vi "Array Functions Part 2.vi"() -> ()   [LabVIEW 2015]
panel:
  out "Initialized + Replaced Result":bool[](array[boolean])
  out "Build Array Result":dbl[](array[numeric])
  out "Array Subset Result":dbl[](array[numeric])
  out "min index(es)":i32
  out "min value":dbl
  out "max index(es)":i32
  out "max value":dbl
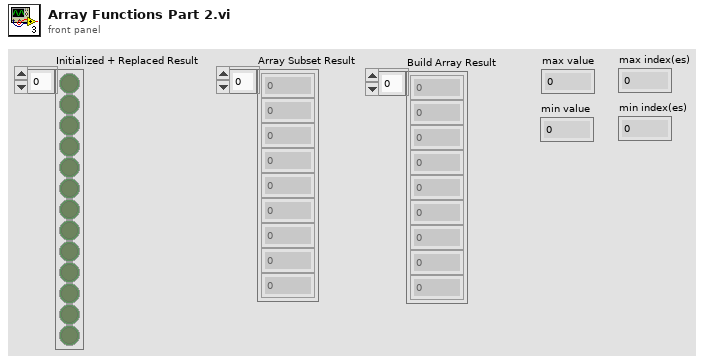
[diagram p1: front panel]
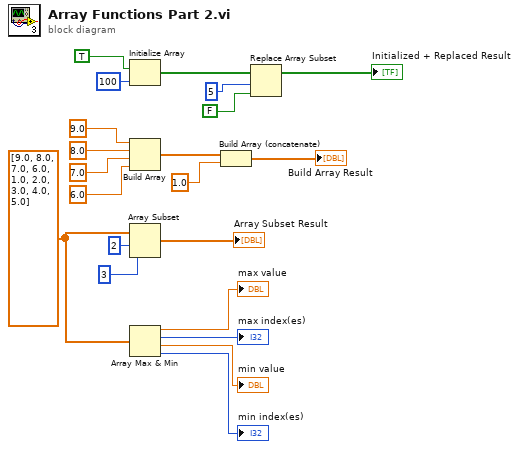
[diagram p0: block diagram]
diagram:
  w17 = dbl[] [9.0, 8.0, 7.0, 6.0, 1.0, 2.0, 3.0, 4.0, 5.0] ("array")
  n1 = Initialize Array "Initialize Array"(TRUE, 100 ("dimension size")) -> (w4:bool[])
  n2 = Build Array "Build Array"(9.0, 8.0, 7.0, 6.0) -> (w8:dbl[])
  n3 = Array Subset "Array Subset"(array=w17, index=2, length=3) -> (→"Array Subset Result":dbl[])
  n4 = Array Max & Min(array=w17) -> (max value=→"max value":dbl, max index (indices)=→"max index(es)":i32, min value=→"min value":dbl, min index (indices)=→"min index(es)":i32)
  n5 = Build Array (concatenate) "Build Array"(w8, 1.0) -> (→"Build Array Result":dbl[])
  n6 = Replace Array Subset "Replace Array Subset"(array=w4, new element=FALSE ("new element/subarray"), index=5) -> (→"Initialized + Replaced Result":bool[])
